vi "NI VeriStand - Set Multiple Channel 2D Array Values.vi"(8 "error in (no error)":errorcluster, 9 "Data Array":T1[](array[typedef]), 10 "Channels":string[](array[string]), 11 "WorkspaceManager in":T2) -> (0 "error out":errorcluster, 3 "WorkspaceManager out":T2)   [LabVIEW 2020, in "NI_VS Workspace ExecutionAPI.lvlib"]
uses:
  <vilib>/NI VeriStand/Execution/Workspace/NI_VS Workspace ExecutionAPI.lvlib
  <vilib>/NI VeriStand/Execution/Workspace/WorkspaceAPI.ctl
  NationalInstruments.VeriStand.ClientAPI
  <vilib>/NI VeriStand/Execution/Workspace/2D Array of Double.ctl
  NationalInstruments.VeriStand
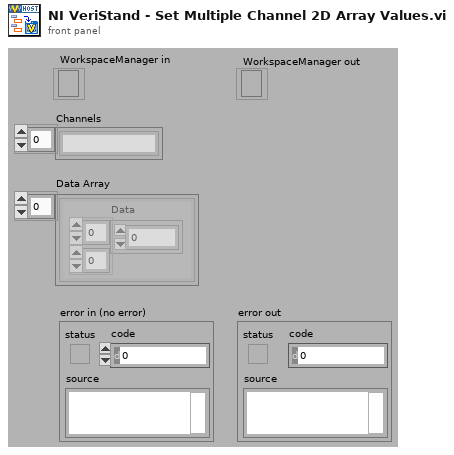
[diagram p1: front panel]
types:
  T1 = typedef "NI_VS Workspace ExecutionAPI.lvlib/2D Array of Double.ctl" = cluster{"Data":dbl[][]}
  T2 = typedef "NI_VS Workspace ExecutionAPI.lvlib/WorkspaceAPI.ctl" = refnum<k24>
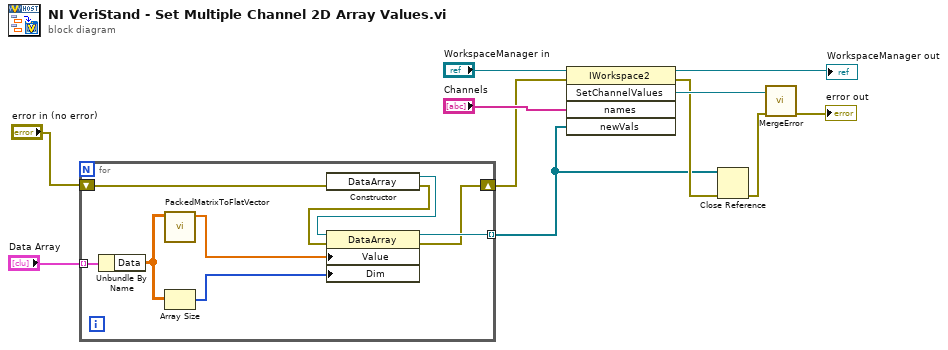
[diagram p0: block diagram]
diagram:
  n1 = for {
    tunnel: [w20] -> w1 mode=indexing
    tunnel: "Data Array" -> [w19] mode=indexing
    shift-right: [w13] -> w4
    shift-left: "error in (no error)" -> [w14]
    n2 = Unbundle By Name(w19) -> ("Data"=w17:dbl[][])
    n3 = call <vilib>:"PackedMatrixToFlatVector.vi"("Matrix"=w17) -> ("FlatVector"=w16:dbl[])  [unwired: 10 in]
    n4 = Array Size(array=w17) -> (size(s)=w18:i32[])
    n5 = constructor class="DataArray"(error in=w14) -> (reference out=w12:refnum<k24>, error out=w15:errorcluster)  [unwired: 2 in, 1 out]
    n6 = property class="DataArray"(reference=w12, error in=w15, "Value"=w16, "Dim"=w18) -> (reference out=w20:refnum<k24>, error out=w13:errorcluster)
  }
  n7 = invoke class="IWorkspace2" method="SetChannelValues"(reference="WorkspaceManager in", error in=w4, "names"="Channels", "newVals"=w1) -> (reference out=→"WorkspaceManager out":T2, error out=w3:errorcluster, "SetChannelValues"=w11:refnum<k24>)  [unwired: 1 in, 2 out]
  n8 = Close Reference(reference=w1, error in (no error)=w3) -> (error out=w2:errorcluster)
  n9 = call <vilib>:"MergeError.vi"("error in (no error)"=w2, "Error"=w11) -> ("error out"=→"error out":errorcluster)  [unwired: 9 out]
